vi "Struct Parse Binary.vi"(8 "error in":errorcluster, 10 "data start offset (0)":i32, 11 "data in":u8[](array[numeric])) -> (0 "error out":errorcluster, 3 "struct items":T1[](array[typedef]))   [LabVIEW 2020, in "GOLPI library.lvlib"]
doc: "Parses binary structure data generated by GNU Octave function 'golpi_conv_struct()' from package GOLPI.\nIt will decode particular struct items into array of items. Each item has type, size, binary data that needs to be later decoded and for arrays of complex data such as array of structs it also returns relative byte offsets of each array cell in the data. \nIf structure contains substruct or array of structs the data needs to be further parsed again by calling this function again with the item data assigned to the data input. If the item was array of structs this function needs to be called for each cell with the cell offset assigned."
uses:
  GOLPI library.lvlib
  Struct Item Record.ctl
  Struct Item Types.ctl
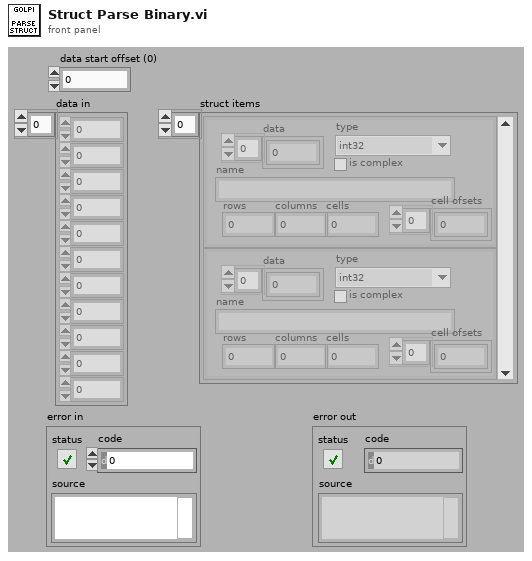
[diagram p1: front panel]
types:
  T1 = typedef "GOLPI library.lvlib/Struct Item Record.ctl" = cluster{"data":u8[], "type":T2, "name":string, "rows":i32, "columns":i32, "cells":i32, "is complex":bool, "cell ofsets":u32[]}
  T2 = typedef "GOLPI library.lvlib/Struct Item Types.ctl" = enum16{"int32", "uint32", "single", "double", "string", "cell array"}
  T3 = enum16{"big-endian, network order", "native, host order", "little-endian"}
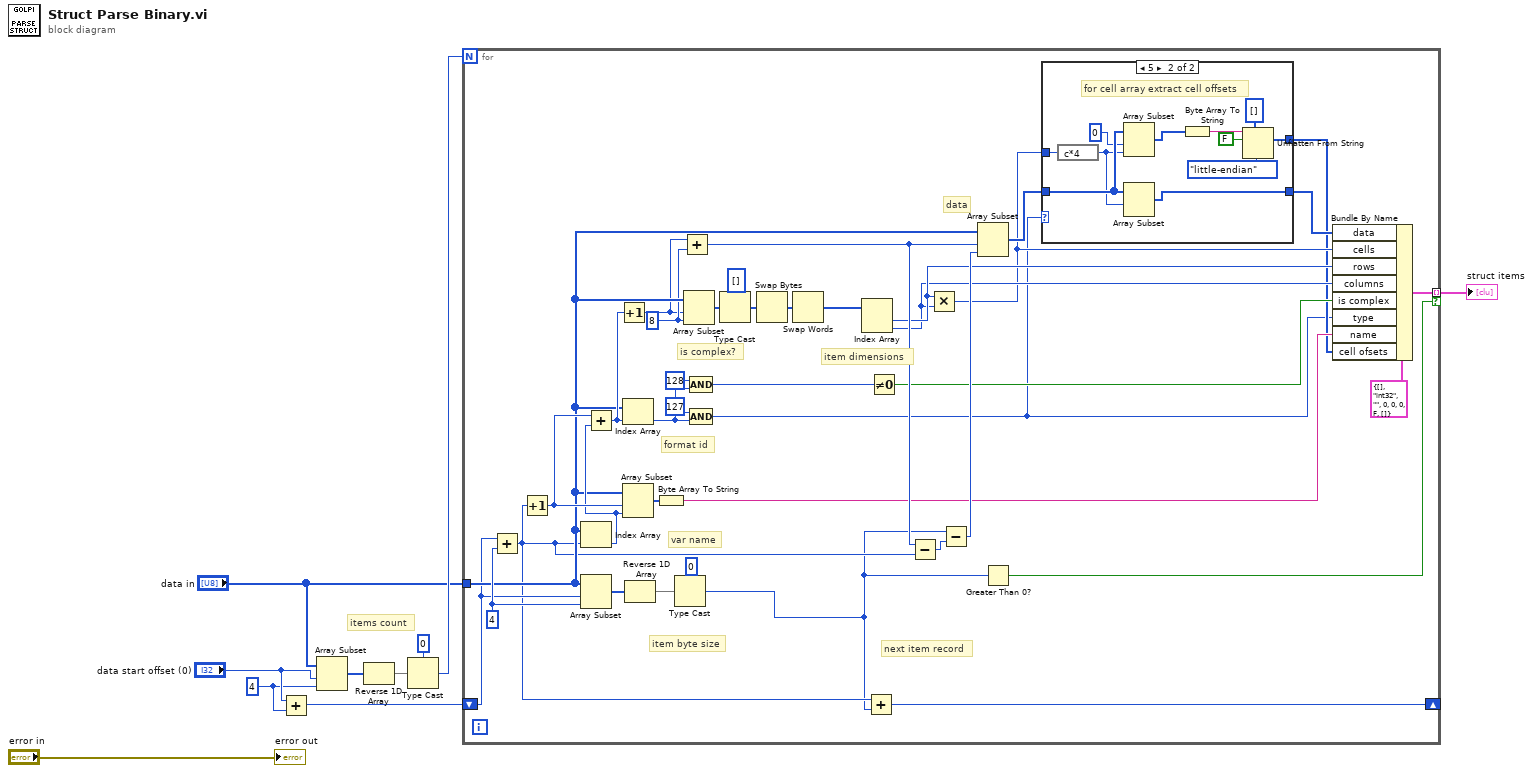
[diagram p0: block diagram]
diagram:
  w2 = 4 ("length")
  # "items count"
  n1 = Add(x="data start offset (0)", y=w2) -> (x+y=w1:i32)
  n2 = Array Subset(array="data in", index="data start offset (0)", length=w2) -> (w5:u8[])
  n3 = Reverse 1D Array(array=w5) -> (reversed array=w10:u8[])
  n4 = Type Cast(type=0, x=w10) -> (*(type *) &x=w8:i32)
  n5 = for {
    N: w8 -> [_]
    tunnel: "data in" -> [w39]
    shift-right: [w31] -> _
    shift-left: w1 -> [w33]
    tunnel: [w24] -> w9 mode=indexing if=w23
    w38 = 8 ("length")
    w47 = 4 ("length")
    # "next item record"
    # "data"
    # "item dimensions"
    # "format id"
    # "is complex?"
    # "var name"
    # "item byte size"
    n6 = Add(x=w33, y=w47) -> (x+y=w32:i32)
    n7 = Increment(x=w32) -> (x+1=w45:i32)
    n8 = Index Array(array=w39, index=w32) -> (element=w44:u8)
    n9 = Array Subset(array=w39, index=w33, length=w47) -> (w48:u8[])
    n10 = Add(x=w45, y=w44) -> (x+y=w40:i32)
    n11 = Increment(x=w40) -> (x+1=w37:i32)
    n12 = Index Array(array=w39, index=w40) -> (element=w42:u8)
    n13 = Array Subset(array=w39, index=w45, length=w44) -> (w46:u8[])
    n14 = Reverse 1D Array(array=w48) -> (reversed array=w22:u8[])
    n15 = Byte Array To String(unsigned byte array=w46) -> (string=w25:string)
    n16 = Type Cast(type=0, x=w22) -> (*(type *) &x=w16:i32)
    n17 = Add(x=w37, y=w38) -> (x+y=w36:i32)
    n18 = Array Subset(array=w39, index=w37, length=w38) -> (w20:u8[])
    n19 = Compound Arithmetic op=AND(u8 128 ("value"), w42) -> (w27:u8)
    n20 = Compound Arithmetic op=AND(u8 127 ("value"), w42) -> (w11:u8)
    n21 = Type Cast(type=i32[] [], x=w20) -> (*(type *) &x=w19:i32[])
    n22 = Swap Bytes(anything=w19) -> (byte swapped=w18:i32[])
    n23 = Swap Words(1:w18) -> (0:w17:i32[])
    n24 = Index Array(array=w17) -> (element #1=w29:i32, element #2=w28:i32)  [unwired: 2 in]
    n25 = Add(x=w32, y=w16) -> (x+y=w31:i32)
    n26 = Not Equal To 0?(x=w27) -> (x != 0?=w26:bool)
    n27 = Subtract(x=w36, y=w32) -> (x-y=w35:i32)
    n28 = Multiply(x=w29, y=w28) -> (x*y=w13:i32)
    n29 = Subtract(x=w16, y=w35) -> (x-y=w34:i32)
    n30 = Array Subset(array=w39, index=w36, length=w34) -> (w15:u8[])
    n31 = Greater Than 0?(x=w16) -> (x > 0?=w23:bool)
    n32 = case shown="5" w11 {
      tunnel: [w50 w58] -> w14
      tunnel: w15 -> [w50 w60]
      tunnel: w13 -> [_ w61]
      tunnel: [_ w55] -> w12
      frame Default {
      }
      frame 5 {
        # "for cell array extract cell offsets"
        n33 = expression code="c*4"(w61) -> (w59:i32)
        n34 = Array Subset(array=w60, index=0, length=w59) -> (w54:u8[])
        n35 = Array Subset(array=w60, index=w59) -> (w58:u8[])  [unwired: 1 in]
        n36 = Byte Array To String(unsigned byte array=w54) -> (string=w53:string)
        n37 = Unflatten From String(type=u32[] [], binary string=w53, data includes array or string size? (T)=FALSE, byte order (0:big-endian, network order)=T3."little-endian") -> (value=w55:u32[])  [unwired: 1 in, 2 out]
      }
    }
    n38 = Bundle By Name(cluster=T1 {"data"=[], "type"=enum."int32", "name"="", "rows"=0, "columns"=0, "cells"=0, "is complex"=FALSE, "cell ofsets"=[]} ("Cluster"), "data"=w14, "cells"=w13, "rows"=w29, "columns"=w28, "is complex"=w26, "type"=w11, "name"=w25, "cell ofsets"=w12) -> (w24:T1)
  }
  "struct items" <- w9
  "error out" <- "error in"
